vi "get reply queue.vi"(8 "error in":errorcluster {"code" format="Error %.0f"}, 11 "NATS Subscription in":refnum<class "NATS Subscription.lvclass">) -> (0 "error out":errorcluster {"code" format="Error %.0f"}, 2 "reply queue":refnum<queue>, 3 "NATS Subscription out":refnum<class "NATS Subscription.lvclass">)   [LabVIEW 2020, in "NATS Subscription.lvlib" / "NATS Subscription.lvclass"]
uses:
  NATS Subscription.lvclass
  NATS Subscription.lvclass/NATS Subscription.ctl
  <vilib>/NATS/NATS Core/Controls/msg type.ctl
  <vilib>/NATS/NATS Core/NATS Core.lvlib
  <vilib>/NATS/NATS Core/Controls/nats message.ctl
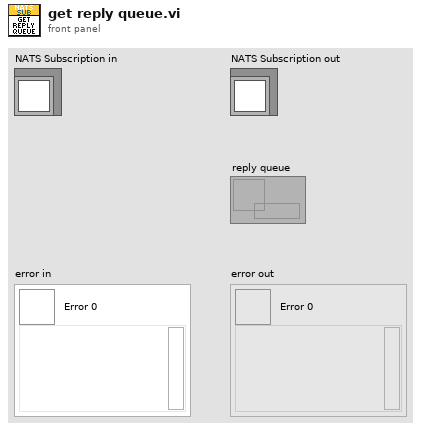
[diagram p1: front panel]
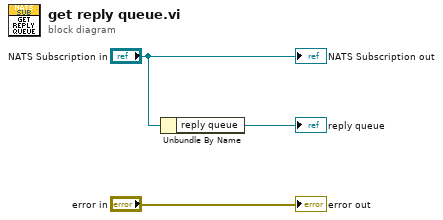
[diagram p0: block diagram]
diagram:
  n1 = Unbundle By Name("NATS Subscription in") -> ("reply queue"=→"reply queue":refnum<queue>)
  "error out" <- "error in"
  "NATS Subscription out" <- "NATS Subscription in"
